vi "Available ini.vi"(8 "error in":errorcluster, 11 "Config file path":path) -> (0 "error out":errorcluster, 1 "Size":i32, 2 "Running":bool[](array[boolean]), 3 "Instances":T1[](array[typedef]), 4 "Select":bool[](array[boolean]), 5 "ini file":path)   [LabVIEW 2015]
uses:
  Instance.ctl
  <vilib>/Utility/config.llb/Read Key (Boolean).vi
  <vilib>/Utility/config.llb/Read Key (String).vi
  <vilib>/Utility/config.llb/NI_LVConfig.lvlib
panel:
  out "index of element":i32
  in  "Cluster":T1
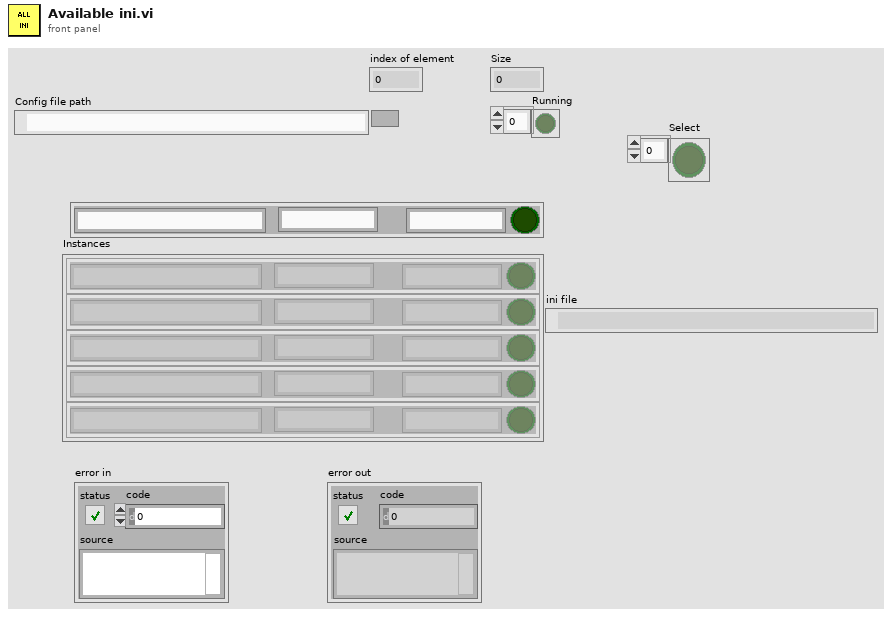
[diagram p1: front panel]
types:
  T1 = typedef "Instance.ctl" = cluster{"Name":string, "Device Name":string, "Running":bool, "File Name":string}
  T2 = typedef "NI_LVConfig.lvlib/Config Data RefNum.ctl" = refnum<k1>
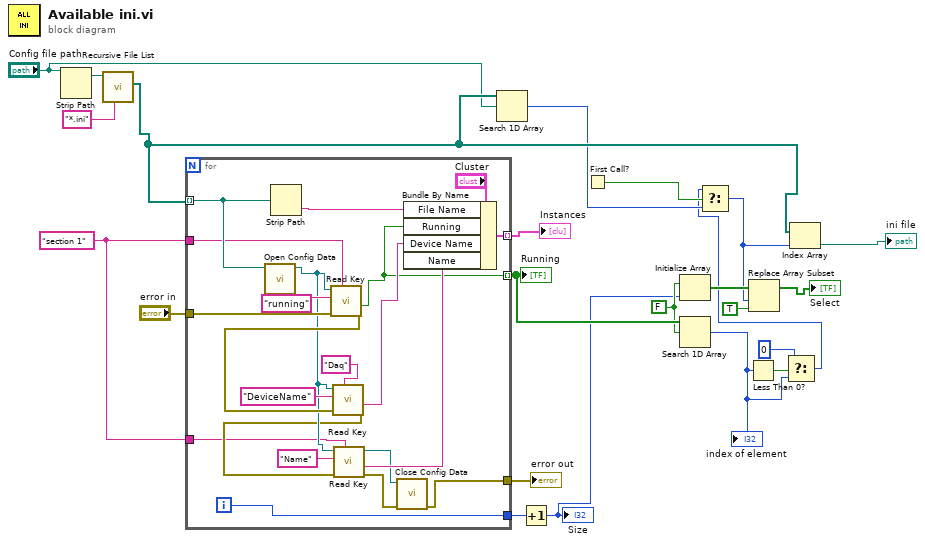
[diagram p0: block diagram]
diagram:
  w12 = "section 1" ("section")
  w18 = FALSE ("element")
  n1 = Strip Path(path="Config file path") -> (stripped path=w13:path)  [unwired: 1 out]
  n2 = call <vilib>:"Recursive File List.vi"("pattern"="*.ini", "Folder Path"=w13) -> ("All Files in Dir"=w10:path[])  [unwired: 5 in, 4 out]
  n3 = for {
    tunnel: w10 -> [w43] mode=indexing
    tunnel: [w35] -> w22 mode=indexing
    tunnel: [w34] -> w19 mode=indexing
    tunnel: [w33] -> w21
    tunnel: "error in" -> [w32]
    tunnel: [w26] -> w20
    tunnel: w12 -> [w25]
    tunnel: w12 -> [w24]
    i -> [w33]
    n4 = call <vilib>:"Open Config Data.vi"("configuration file path"=w43) -> ("refnum"=w30:T2)  [unwired: 8 in, 2 out]
    n5 = Strip Path(path=w43) -> (name=w44:string)  [unwired: 1 out]
    n6 = call-poly <vilib>:"Read Key.vi"("section"=w25, "error in (no error)"=w32, "key"="running", "refnum"=w30) -> ("error out"=w31:errorcluster, "value"=w34:bool)  [unwired: 4 in, 2 out]
    n7 = call-poly <vilib>:"Read Key.vi"("section"="Daq", "error in (no error)"=w31, "key"="DeviceName", "refnum"=w30) -> ("error out"=w29:errorcluster, "value"=w38:string)  [unwired: 4 in, 2 out]
    n8 = call-poly <vilib>:"Read Key.vi"("section"=w24, "error in (no error)"=w29, "key"="Name", "refnum"=w30) -> ("error out"=w28:errorcluster, "value"=w37:string, "refnum out"=w36:T2)  [unwired: 4 in, 1 out]
    n9 = call <vilib>:"Close Config Data.vi"("error in (no error)"=w28, "refnum"=w36) -> ("error out"=w26:errorcluster)  [unwired: 8 in, 1 out]
    n10 = Bundle By Name(cluster="Cluster", "File Name"=w44, "Running"=w34, "Device Name"=w38, "Name"=w37) -> (w35:T1)
  }
  "Instances" <- w22
  "error out" <- w20
  "Running" <- w19
  n11 = Search 1D Array(1D array=w10, element="Config file path") -> (index of element=w7:i32)  [unwired: 1 in]
  n12 = Increment(x=w21) -> (x+1=w8:i32)
  "Size" <- w8
  n13 = First Call?() -> (First Call?: T/F=w11:bool)
  n14 = Initialize Array(w18, w8) -> (w17:bool[])
  n15 = Search 1D Array(1D array=w19, element=w18) -> (index of element=w3:i32)  [unwired: 1 in]
  "index of element" <- w3
  n16 = Less Than 0?(x=w3) -> (x < 0?=w4:bool)
  n17 = Select(t=0, s=w4, f=w3) -> (s? t:f=w2:i32)
  n18 = Select(t=w2, s=w11, f=w7) -> (s? t:f=w6:i32)
  n19 = Replace Array Subset(array=w17, new element=TRUE ("new element/subarray"), index=w6) -> (→"Select":bool[])
  n20 = Index Array(array=w10, index=w6) -> (element=→"ini file":path)
